vi "pp2_DAQinit.vi"(8 "error in (no error)":errorcluster, 11 "Daq config in":T1={"Sound AO"="Dev3/ao0", "Shock intesity AO"="Dev3/ao1", "Code_LED DO"="Dev3/port1:2", "Switch DI"="Dev3/port2/line0:1", "Webcam"="cam9", "Sound AO task"="", "Sound card task"=0, "Shock intensity AO task"="", "Code_LED DO task"="", "Switch DI task"="", "AO <=> Sound card"=FALSE, "Sound card"=0, "sample rate"=100000.0, "Variable shock"=FALSE, "Webcam on"=FALSE, "Tone gate PFI"="/Dev3/PFI1", "Waveform memo"={"t0"=timestamp(0 s since 1904-01-01), "dt"=1.0, "Y"=[]}, "First time"=FALSE} {"sample rate" min=8000.0; "Sound card task" format="%.0x"}) -> (0 "error out":errorcluster, 3 "Daq config out":T1={"Sound AO"="Dev2/ao0", "Shock intesity AO"="Dev1/ao1", "Code_LED DO"="Dev1/port1:2", "Switch DI"="Dev1/port0/line0:1", "Webcam"="cam0", "Sound AO task"="", "Sound card task"=0, "Shock intensity AO task"="", "Code_LED DO task"="", "Switch DI task"="", "AO <=> Sound card"=FALSE, "Sound card"=0, "sample rate"=8000.0, "Variable shock"=FALSE, "Webcam on"=FALSE, "Tone gate PFI"="/Dev1/PFI1", "Waveform memo"={"t0"=timestamp(0 s since 1904-01-01), "dt"=1.0, "Y"=[]}, "First time"=FALSE} {"sample rate" min=8000.0; "Sound card task" format="%.0x"})   [LabVIEW 2013]
uses:
  pp2_CTL_DaqConfig.ctl
  <vilib>/userdefined/High Color/IMAQdx.ctl
  <vilib>/sound2/lvsound2.llb/Sound Output Task ID.ctl
  <vilib>/sound2/lvsound2.llb/Sampling Mode.ctl
  <vilib>/sound2/lvsound2.llb/Sound Data Format.ctl
  <vilib>/DAQmx/create/channels.llb/DAQmx Create Channel (DO-Digital Output).vi
  <vilib>/DAQmx/create/channels.llb/DAQmx Create Channel (DI-Digital Input).vi
  <vilib>/DAQmx/create/channels.llb/DAQmx Create Channel (AO-Voltage-Basic).vi
  <vilib>/DAQmx/configure/timing.llb/DAQmx Timing (Sample Clock).vi
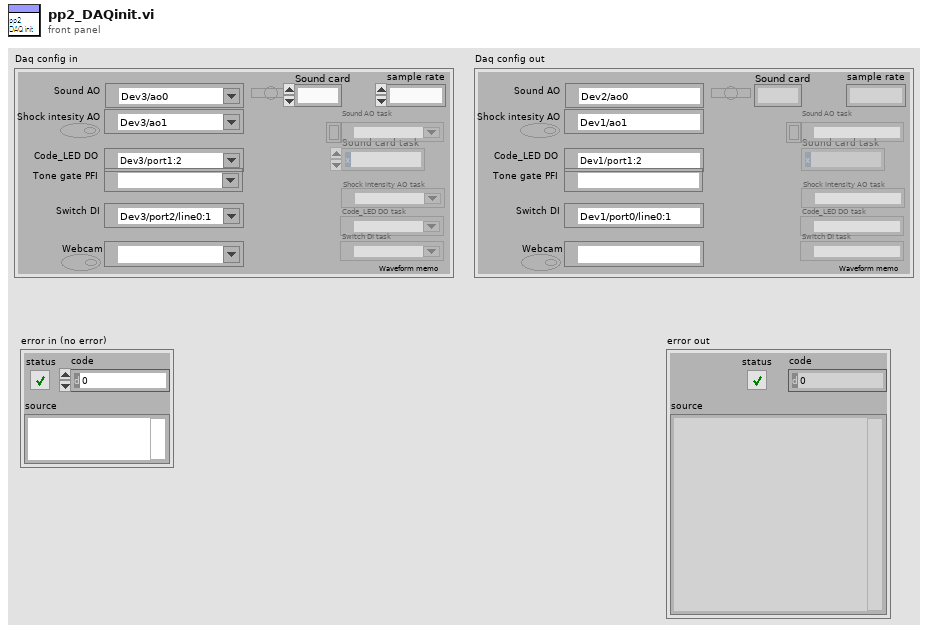
[diagram p1: front panel]
types:
  T1 = typedef "pp2_CTL_DaqConfig.ctl" = cluster{"Sound AO":tag, "Shock intesity AO":tag, "Code_LED DO":tag, "Switch DI":tag, "Webcam":T2, "Sound AO task":refnum<k21>, "Sound card task":T3, "Shock intensity AO task":refnum<k21>, "Code_LED DO task":refnum<k21>, "Switch DI task":refnum<k21>, "AO <=> Sound card":bool, "Sound card":u32, "sample rate":dbl, "Variable shock":bool, "Webcam on":bool, "Tone gate PFI":tag, "Waveform memo":waveform(dbl), "First time":bool}
  T2 = typedef "IMAQdx.ctl" = refnum<k21>
  T3 = typedef "Sound Output Task ID.ctl" = u32
  T4 = typedef "Sound Data Format.ctl" = cluster{"sample rate (S/s)":dbl, "number of channels":i32, "bits per sample":i32}
  T5 = typedef "Sampling Mode.ctl" = i32
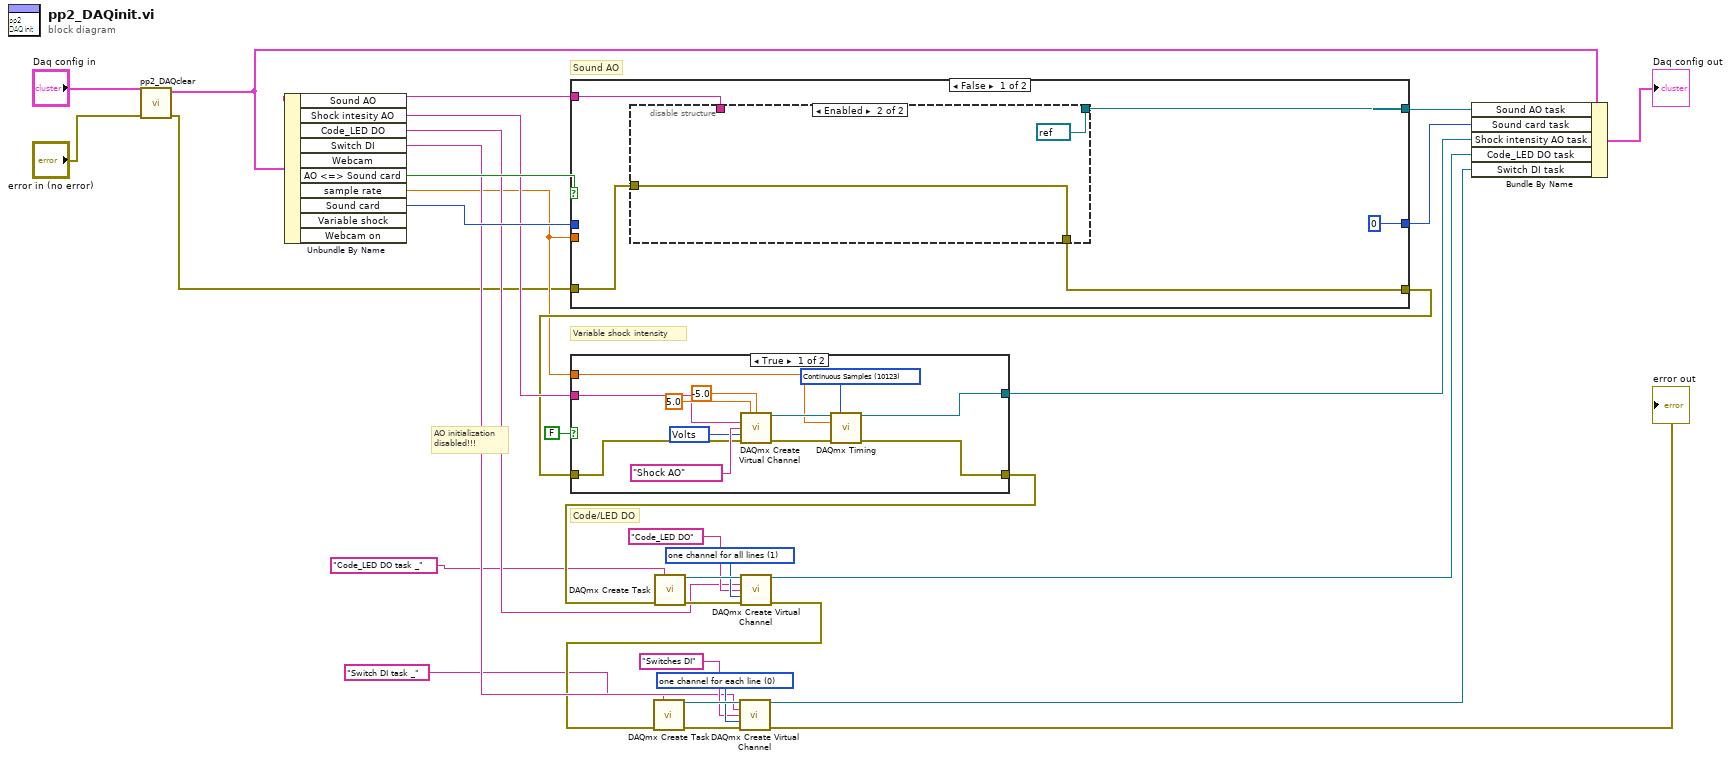
[diagram p0: block diagram]
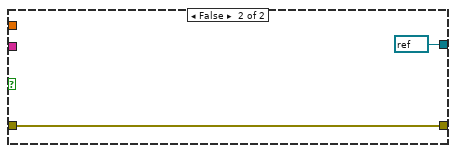
[diagram p2: hidden frame]
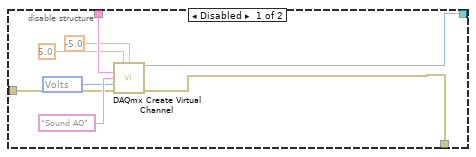
[diagram p3: hidden frame]
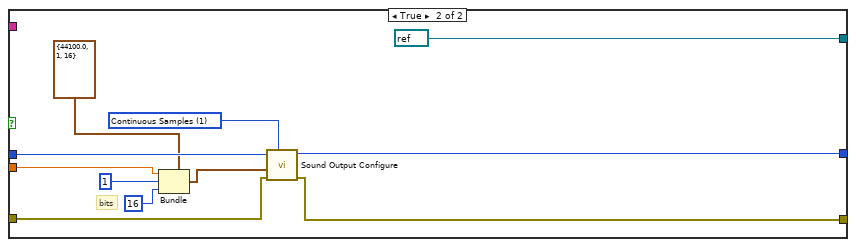
[diagram p4: hidden frame]
diagram:
  w17 = 0 items=["one channel for each line", "one channel for all lines"] ("line grouping")
  w22 = 1 items=["one channel for each line", "one channel for all lines"] ("line grouping")
  # "AO initialization\ndisabled!!!"
  # "Code/LED DO"
  # "Variable shock intensity"
  # "Sound AO"
  n1 = call "pp2_DAQclear.vi"("error in (no error)"="error in (no error)", "Daq config in"="Daq config in") -> ("error out"=w4:errorcluster, "Daq config out"=w6:T1)  [unwired: 8 in]
  n2 = Unbundle By Name(w6) -> ("Sound AO"=w31:tag, "Shock intesity AO"=w26:tag, "Code_LED DO"=w20:tag, "Switch DI"=w15:tag, "AO <=> Sound card"=w32:bool, "sample rate"=w8:dbl, "Sound card"=w28:u32)  [unwired: 3 out]
  n3 = case shown="False" w32 {
    tunnel: w31 -> [w37 _]
    tunnel: [w35 refnum<k21> refnum ("task out")] -> w29
    tunnel: w28 -> [_ w57]
    tunnel: [T3 0 ("task ID") w53] -> w27
    tunnel: w4 -> [w33 w52]
    tunnel: [w34 w51] -> w12
    tunnel: w8 -> [_ w50]
    frame False {
      n4 = disable-structure shown="Enabled" {
        disable-tunnel: w37 -> [w45 _]
        disable-tunnel: [w40 refnum<k21> refnum ("task out")] -> w35
        disable-tunnel: [w39 w46] -> w34
        disable-tunnel: w33 -> [w38 w46]
        frame Disabled {
          w41 = 10348 items=["Volts"=10348, "From Custom Scale"=10065] ("units")
          n5 = call-poly <vilib>:"DAQmx Create Virtual Channel.vi"("maximum value"=5.0, "minimum value"=-5.0, "physical channels"=w45, "name to assign"="Sound AO", "units"=w41, "error in"=w38) -> ("task out"=w40:refnum<k21>, "error out"=w39:errorcluster)  [unwired: 8 in]
        }
        frame Enabled {
        }
      }
    }
    frame True {
      w56 = T5 1 items=["Finite Samples", "Continuous Samples"] ("sample mode")
      # "bits"
      n6 = Bundle(cluster=T4 {"sample rate (S/s)"=44100.0, "number of channels"=1, "bits per sample"=16} ("sound format"), "sample rate (S/s)"=w50, "number of channels"=1 ("Input.BufSize"), "bits per sample"=16 ("Input.BufSize")) -> (w48:T4)
      n7 = call <vilib>:"Sound Output Configure.vi"("sample mode"=w56, "error in (no error)"=w52, "sound format"=w48, "device ID"=w57) -> ("error out"=w51:errorcluster, "task ID"=w53:T3)  [unwired: 6 in]
    }
  }
  n8 = case shown="True" FALSE {
    tunnel: w26 -> [w67 _]
    tunnel: [w60 refnum<k21> refnum ("task out")] -> w25
    tunnel: w8 -> [w63 _]
    tunnel: w12 -> [w61 w72]
    tunnel: [w59 w72] -> w11
    frame True {
      w62 = 10123 items=["Finite Samples"=10178, "Continuous Samples"=10123, "Hardware Timed Single Point"=12522] ("sample mode")
      w68 = 10348 items=["Volts"=10348, "From Custom Scale"=10065] ("units")
      n9 = call-poly <vilib>:"DAQmx Create Virtual Channel.vi"("maximum value"=5.0, "minimum value"=-5.0, "physical channels"=w67, "name to assign"="Shock AO", "units"=w68, "error in"=w61) -> ("task out"=w65:refnum<k21>, "error out"=w64:errorcluster)  [unwired: 8 in]
      n10 = call-poly <vilib>:"DAQmx Timing.vi"("task/channels in"=w65, "sample mode"=w62, "rate"=w63, "error in"=w64) -> ("task out"=w60:refnum<k21>, "error out"=w59:errorcluster)  [unwired: 10 in]
    }
    frame False {
    }
  }
  n11 = call <vilib>:"DAQmx Create Task.vi"("new task name"="Code_LED DO task _", "error in"=w11) -> ("task out"=w23:refnum<k21>, "error out"=w24:errorcluster)  [unwired: 12 in]
  n12 = call-poly <vilib>:"DAQmx Create Virtual Channel.vi"("task in"=w23, "lines"=w20, "name to assign"="Code_LED DO", "line grouping"=w22, "error in"=w24) -> ("task out"=w14:refnum<k21>, "error out"=w10:errorcluster)  [unwired: 9 in]
  n13 = call <vilib>:"DAQmx Create Task.vi"("new task name"="Switch DI task _", "error in"=w10) -> ("task out"=w18:refnum<k21>, "error out"=w19:errorcluster)  [unwired: 12 in]
  n14 = call-poly <vilib>:"DAQmx Create Virtual Channel.vi"("task in"=w18, "lines"=w15, "name to assign"="Switches DI", "line grouping"=w17, "error in"=w19) -> ("task out"=w13:refnum<k21>, "error out"=→"error out":errorcluster)  [unwired: 9 in]
  n15 = Bundle By Name(cluster=w6, "Sound AO task"=w29, "Sound card task"=w27, "Shock intensity AO task"=w25, "Code_LED DO task"=w14, "Switch DI task"=w13) -> (→"Daq config out":T1)
